vi "Arduino Write Int.vi"(7 "Command":string, 8 "error in (no error)":errorcluster, 9 "Data":u32, 11 "COM Port In":refnum<visa-resource-name>) -> (0 "error out":errorcluster, 3 "COM Port Out":refnum<visa-resource-name>)   [LabVIEW 2023, in "Arduino DAQ.lvlib"]
uses:
  Arduino DAQ.lvlib
panel:
  out "response":string
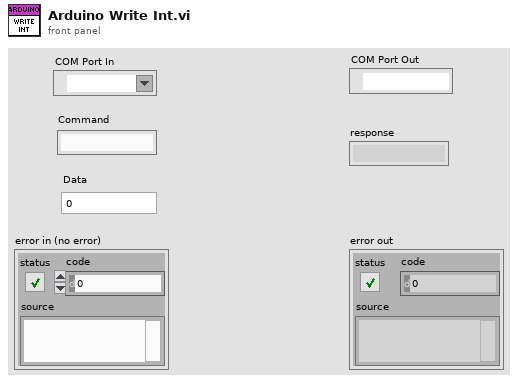
[diagram p1: front panel]
types:
  T1 = enum16{"big-endian, network order", "native, host order", "little-endian"}
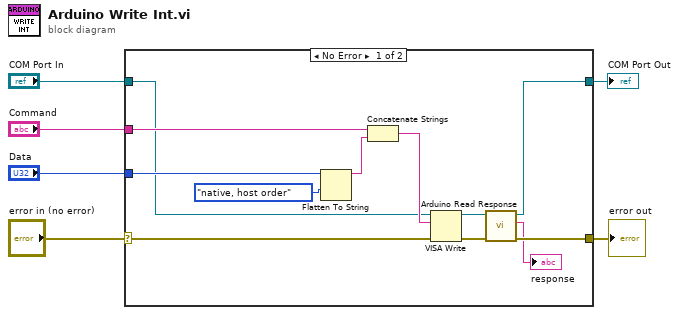
[diagram p0: block diagram]
diagram:
  n1 = case shown="No Error" "error in (no error)" {
    selector: "error in (no error)" -> [w11 w20]
    tunnel: [w13 w20] -> w6
    tunnel: "COM Port In" -> [w12 w19]
    tunnel: "Command" -> [w18 _]
    tunnel: [w8 w19] -> w2
    tunnel: "Data" -> [w16 _]
    frame No Error {
      n2 = Flatten To String(anything=w16, byte order (0:big-endian, network order)=T1."native, host order") -> (data string=w14:string)  [unwired: 2 in, 2 out]
      n3 = Concatenate Strings(w18, w14) -> (w17:string)
      n4 = VISA Write(VISA resource name=w12, write buffer=w17, error in (no error)=w11) -> (VISA resource name out=w10:refnum<visa-resource-name>, error out=w9:errorcluster)  [unwired: 1 out]
      n5 = call "Arduino Read Response.vi"("error in"=w9, "COM Port In"=w10) -> ("error out"=w13:errorcluster, "response"=→"response":string, "COM Port Out 2"=w8:refnum<visa-resource-name>)  [unwired: 7 in]
    }
    frame Error {
    }
  }
  "error out" <- w6
  "COM Port Out" <- w2
